vi "WaitForInitialize.vi"(3 "error in (no error)":errorcluster) -> (1 "error out":errorcluster)   [LabVIEW 2009]
doc: "This VI is the solution to Exercise 3-1 of the LabVIEW Basics II course.\n\nThis VI will accept a user name and password, and after the OK button is pressed, verify if the information is valid using the Verify Information subVI. The name and password controls are initialized to empty strings and the Key Focus attribute of the Login Name control is set to TRUE.\n\nYou will use this VI in Application Exercise.vi (Exercise 5-1) as your login screen."
panel:
  in  "stop":bool
  # "Waitting for initialization to complete"
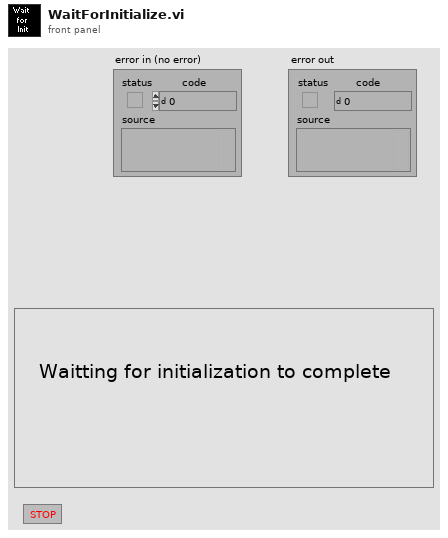
[diagram p1: front panel]
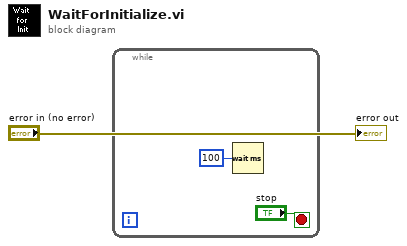
[diagram p0: block diagram]
diagram:
  n1 = while {
    stop <- "stop" stop-if-true
    n2 = Wait (ms)(milliseconds to wait=u32 100) -> ()  [unwired: 1 out]
  }
  "error out" <- "error in (no error)"
